vi "DownConvert Test Node.vi"(10 "Test Node (Extended)":T3) -> (2 "Test Node":T1)   [LabVIEW 2013, in "Caraya.lvlib" / "Test Result.lvclass"]
uses:
  Test Result.lvclass
  Test Node (Extended).ctl
  Test Registration Data.ctl
  Test Node.ctl
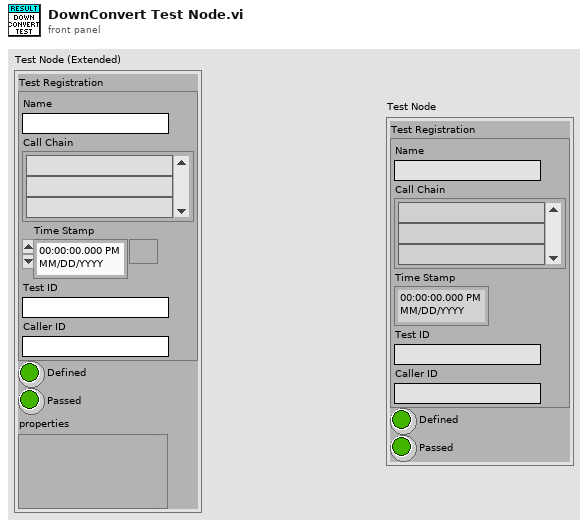
[diagram p1: front panel]
types:
  T1 = typedef "Caraya.lvlib/Test Result.lvclass/Test Node.ctl" = cluster{"Test Registration":T2, "Defined":bool, "Passed":bool}
  T2 = typedef "Caraya.lvlib/Test Result.lvclass/Test Registration Data.ctl" = cluster{"Name":string, "Call Chain":string[], "Time Stamp":timestamp, "Test ID":string, "Caller ID":string}
  T3 = typedef "Caraya.lvlib/Test Result.lvclass/Test Node (Extended).ctl" = cluster{"Test Registration":T2, "Defined":bool, "Passed":bool, "properties":variant}
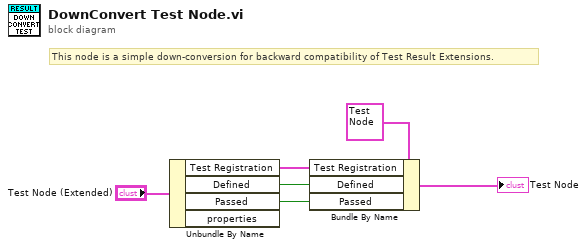
[diagram p0: block diagram]
diagram:
  # "This node is a simple down-conversion for backward compatibility of Test Result Extensions."
  n1 = Unbundle By Name("Test Node (Extended)") -> ("Test Registration"=w3:T2, "Defined"=w2:bool, "Passed"=w1:bool)  [unwired: 1 out]
  n2 = Bundle By Name(cluster=T1 {"Test Registration"={"Name"="", "Call Chain"=[], "Time Stamp"=timestamp(0 s since 1904-01-01), "Test ID"="", "Caller ID"=""}, "Defined"=FALSE, "Passed"=FALSE} ("Test Node"), "Test Registration"=w3, "Defined"=w2, "Passed"=w1) -> (→"Test Node":T1)
